vi "Inverse_Auto_Amp_Spectra.vi"(8 "df":dbl, 9 "t":dbl[](array[numeric]), 10 "Amp Spectrum Mag (Vrms)":dbl[](array[numeric]), 11 "Amp Spectrum Phase (radians)":dbl[](array[numeric])) -> (0 "dt":dbl, 3 "X":dbl[](array[numeric]))   [LabVIEW 2012]
uses:
  <vilib>/Analysis/2dsp.llb/Inverse Real FFT.vi
  <vilib>/Analysis/1siggen.llb/Ramp Pattern by Samples.vi
  <vilib>/Analysis/NI_AALPro.lvlib
  <vilib>/Analysis/NI_AALBase.lvlib
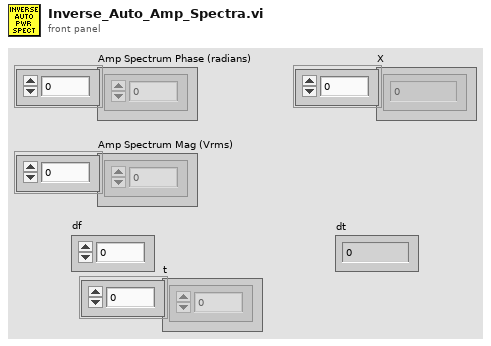
[diagram p1: front panel]
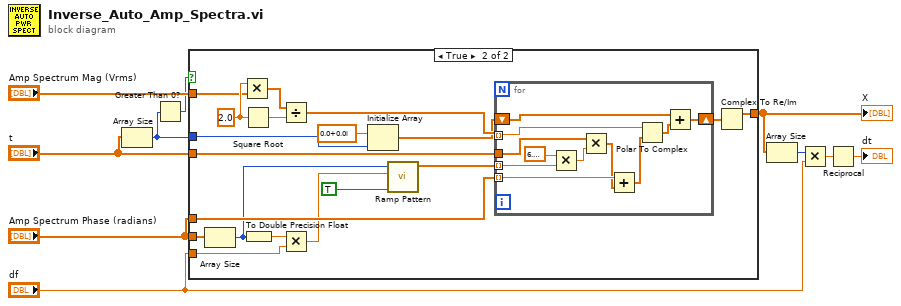
[diagram p0: block diagram]
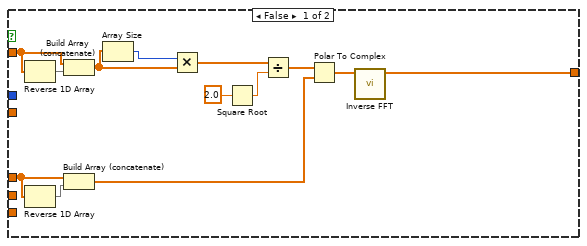
[diagram p2: hidden frame]
diagram:
  n1 = Array Size(array="t") -> (size(s)=w4:i32)
  n2 = Greater Than 0?(x=w4) -> (x > 0?=w5:bool)
  n3 = case shown="True" w5 {
    tunnel: "Amp Spectrum Phase (radians)" -> [w14 w37]
    tunnel: "Amp Spectrum Mag (Vrms)" -> [w12 w39]
    tunnel: [w11 w25] -> w9
    tunnel: w4 -> [_ w27]
    tunnel: "t" -> [_ w33]
    tunnel: "Amp Spectrum Phase (radians)" -> [_ w30]
    tunnel: "df" -> [_ w29]
    frame False {
      n4 = Reverse 1D Array(array=w12) -> (reversed array=w23:dbl[])
      n5 = Reverse 1D Array(array=w14) -> (reversed array=w22:dbl[])
      n6 = Build Array (concatenate)(w12, w23) -> (w13:dbl[])
      n7 = Build Array (concatenate)(w14, w22) -> (w16:dbl[])
      n8 = Array Size(array=w13) -> (size(s)=w17:i32)
      n9 = Multiply(x=w17, y=w13) -> (x*y=w18:dbl[])
      n10 = Square Root(x=2.0) -> (sqrt(x)=w19:dbl)
      n11 = Divide(x=w18, y=w19) -> (x/y=w21:dbl[])
      n12 = Polar To Complex(1:w16, 2:w21) -> (0:w15:cdb[])
      n13 = call-poly <vilib>:"Inverse FFT.vi"("FFT {X}"=w15) -> ("X"=w11:dbl[])  [unwired: 9 in, 1 out]
    }
    frame True {
      w41 = 2.0 ("x")
      n14 = Array Size(array=w30) -> (size(s)=w24:i32)
      n15 = Multiply(x=w41, y=w39) -> (x*y=w40:dbl[])
      n16 = Square Root(x=w41) -> (sqrt(x)=w42:dbl)
      n17 = To Double Precision Float(number=w24) -> (double precision float=w32:dbl)
      n18 = Divide(x=w40, y=w42) -> (x/y=w38:dbl[])
      n19 = Multiply(x=w32, y=w29) -> (x*y=w31:dbl)
      n20 = Initialize Array(cdb 0.0+0.0i ("element"), w27) -> (w34:cdb[])
      n21 = call-poly <vilib>:"Ramp Pattern.vi"("exclude end?"=TRUE, "end"=w31, "samples"=w24) -> ("Ramp Pattern"=w26:dbl[])  [unwired: 7 in, 1 out]
      n22 = for {
        tunnel: w38 -> [w51] mode=indexing
        tunnel: w37 -> [w53] mode=indexing
        tunnel: w33 -> [w47]
        tunnel: w26 -> [w50] mode=indexing
        shift-right: [w45] -> w36
        shift-left: w34 -> [w43]
        n23 = Multiply(x=6.283185307179586, y=w50) -> (x*y=w48:dbl)
        n24 = Multiply(x=w47, y=w48) -> (x*y=w46:dbl[])
        n25 = Add(x=w53, y=w46) -> (x+y=w52:dbl[])
        n26 = Polar To Complex(1:w52, 2:w51) -> (0:w44:cdb[])
        n27 = Add(x=w43, y=w44) -> (x+y=w45:cdb[])
      }
      n28 = Complex To Re/Im(x + iy=w36) -> (x=w25:dbl[])  [unwired: 1 out]
    }
  }
  "X" <- w9
  n29 = Array Size(array=w9) -> (size(s)=w7:i32)
  n30 = Multiply(x=w7, y="df") -> (x*y=w8:dbl)
  n31 = Reciprocal(x=w8) -> (1/x=→"dt":dbl)
